vi "CalculateLensThickness.vi"(9 "Refractive index":dbl, 10 "Measurement Peak Position":dbl, 11 "Callibration Peak Position":dbl) -> (3 "Lens thickness":dbl)   [LabVIEW 2013]
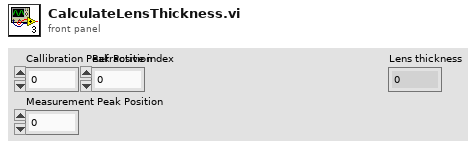
[diagram p1: front panel]
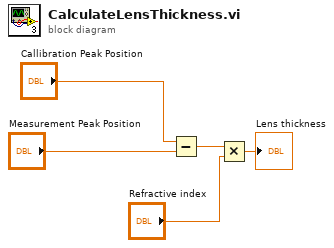
[diagram p0: block diagram]
diagram:
  n1 = Subtract(x="Callibration Peak Position", y="Measurement Peak Position") -> (x-y=w5:dbl)
  n2 = Multiply(x=w5, y="Refractive index") -> (x*y=→"Lens thickness":dbl)
